vi "6-8.vi"() -> ()   [LabVIEW 2017]
panel:
  out "Waveform Chart":dbl(graph)
  in  "access (0:read/write)":enum16{"read/write", "read-only", "write-only"}(ring)
  in  "operation (0:open)":T1(ring)
  in  "file path (use dialog)":path
  in  "stop":bool
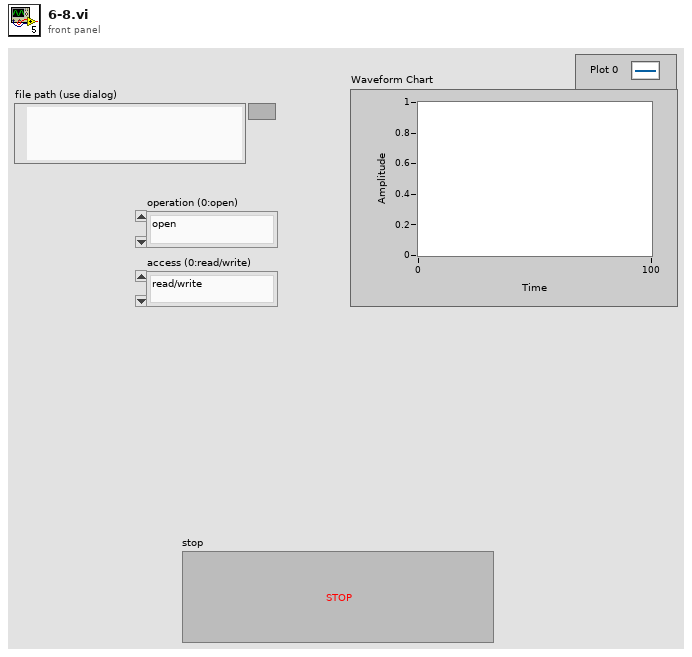
[diagram p1: front panel]
types:
  T1 = enum16{"open", "replace", "create", "open or create", "replace or create", "replace or create with confirmation"}
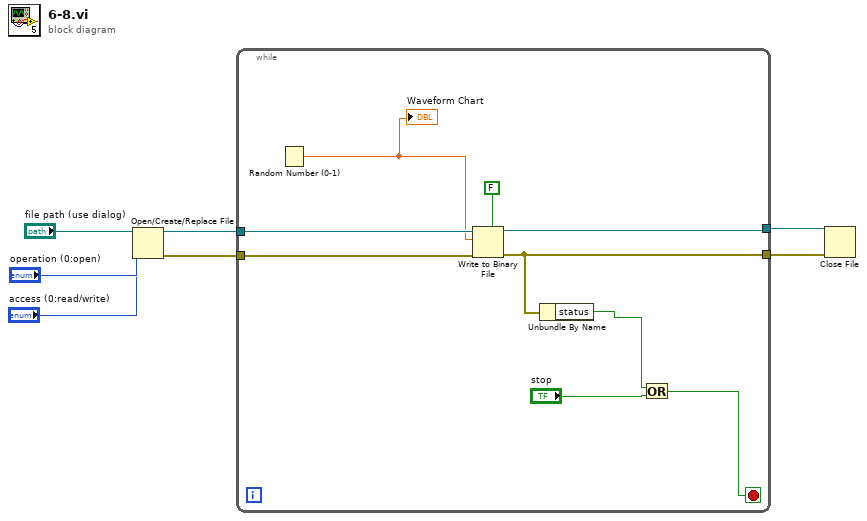
[diagram p0: block diagram]
diagram:
  n1 = Open/Create/Replace File(file path (use dialog)="file path (use dialog)", operation (0:open)="operation (0:open)", access (0:read/write)="access (0:read/write)") -> (refnum out=w7:refnum<file>, error out=w6:errorcluster)  [unwired: 3 in, 1 out]
  n2 = while {
    tunnel: w7 -> [w16]
    tunnel: w6 -> [w15]
    tunnel: [w11] -> w1
    tunnel: [w12] -> w2
    stop <- w8 stop-if-true
    n3 = Random Number (0-1)() -> (number: 0 to 1=w13:dbl)
    "Waveform Chart" <- w13
    n4 = Write to Binary File(file (use dialog)=w16, data=w13, error in=w15, 5:FALSE ("prepend array or string size? (T)")) -> (refnum out=w12:refnum<file>, error out=w11:errorcluster)  [unwired: 2 in, 1 out]
    n5 = Unbundle By Name(w11) -> ("status"=w10:bool)
    n6 = Or(x=w10, y="stop") -> (x .or. y?=w8:bool)
  }
  n7 = Close File(refnum=w2, error in=w1) -> ()  [unwired: 2 out]
